vi "testingUpdateGains.vi"(10 "AdmittanceCoeffs":T1, 11 "PID gains":T2) -> (2 "AdmittanceCoeffs":T1, 3 "PID gains":T2={"proportional gain (Kc)"=1.0, "integral time (Ti, min)"=0.01, "derivative time (Td, min)"=0.0})   [LabVIEW 2016, in "controllerLibrary.lvlib"]
uses:
  controllerLibrary.lvlib
  Controls/AdmittanceGains.ctl
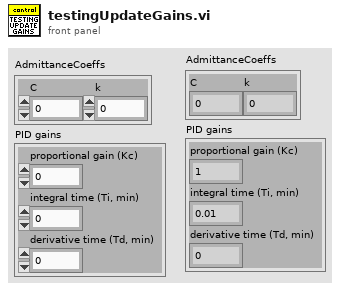
[diagram p1: front panel]
types:
  T1 = typedef "controllerLibrary.lvlib/AdmittanceGains.ctl" = cluster{"C":dbl, "k":dbl}
  T2 = cluster{"proportional gain (Kc)":dbl, "integral time (Ti, min)":dbl, "derivative time (Td, min)":dbl}
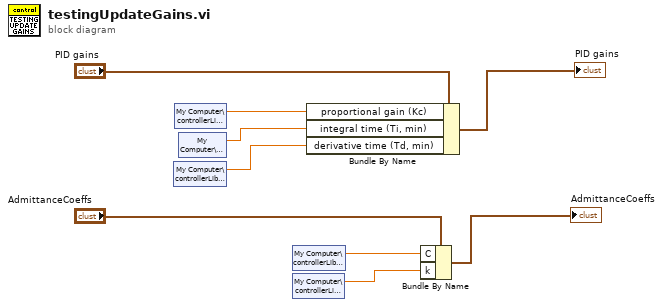
[diagram p0: block diagram]
diagram:
  n1 = shared-variable "My Computer\\controllerLibrary.lvlib\\D"() -> (w1:dbl)  [unwired: 1 in, 1 out]
  n2 = shared-variable "My Computer\\controllerLibrary.lvlib\\P"() -> (w3:dbl)  [unwired: 1 in, 1 out]
  n3 = shared-variable "My Computer\\controllerLibrary.lvlib\\I"() -> (w2:dbl)  [unwired: 1 in, 1 out]
  n4 = shared-variable "My Computer\\controllerLibrary.lvlib\\C"() -> (w5:dbl)  [unwired: 1 in, 1 out]
  n5 = shared-variable "My Computer\\controllerLibrary.lvlib\\K"() -> (w4:dbl)  [unwired: 1 in, 1 out]
  n6 = Bundle By Name(cluster="PID gains", "proportional gain (Kc)"=w3, "integral time (Ti, min)"=w2, "derivative time (Td, min)"=w1) -> (→"PID gains":T2)
  n7 = Bundle By Name(cluster="AdmittanceCoeffs", "C"=w5, "k"=w4) -> (→"AdmittanceCoeffs":T1)
